vi "DOFreq.vi"(6 "Slot":T1, 8 "error in":errorcluster, 10 "State":string, 11 "CH":string) -> (0 "error out":errorcluster)   [LabVIEW 2013]
uses:
  SystemCode/SysControl/Slot.ctl
  <vilib>/DAQmx/write.llb/DAQmx Write (Digital Bool 1Line 1Point).vi
  SourceCode/GlobalValue.vi
  <vilib>/DAQmx/create/channels.llb/DAQmx Create Channel (DO-Digital Output).vi
  <vilib>/DAQmx/miscellaneous.llb/DAQmx Fill In Error Info.vi
panel:
  out "Line/port":tag="PCI-6229/port0/line0:1"
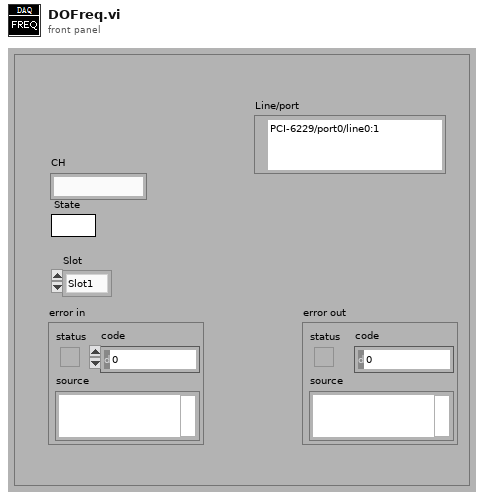
[diagram p1: front panel]
types:
  T1 = typedef "Slot.ctl" = enum16{"Slot1", "Slot2", "Slot3", "Slot4"}
  T2 = typedef "DAQConfig.ctl" = cluster{"DIO":string[][], "AO":string[][], "AI":string[][]}
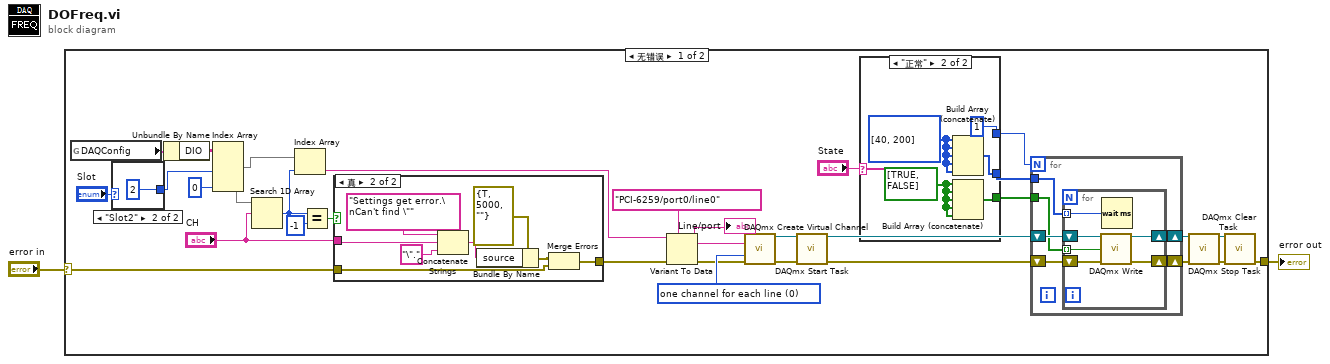
[diagram p0: block diagram]
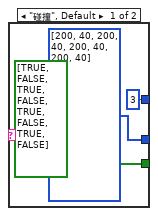
[diagram p2: hidden frame]
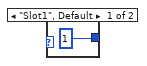
[diagram p3: hidden frame]
diagram:
  n1 = case shown="无错误" "error in" {
    selector: "error in" -> [w22 w65]
    tunnel: [w30 w65] -> w2
    frame No Error {
      w12 = 0 items=["one channel for each line", "one channel for all lines"] ("line grouping")
      n2 = global read "GlobalValue.vi" "DAQConfig"() -> (w19:T2)
      n3 = case shown="\"Slot2\"" "Slot" {
        tunnel: [1 ("索引 (行)") 2 ("索引 (行)")] -> w20
        frame "Slot1", Default {
        }
        frame "Slot2" {
        }
      }
      n4 = Unbundle By Name(w19) -> ("DIO"=w32:string[][])
      n5 = Index Array(array=w32, index (col) #1=w20, index (col) #2=0 ("索引 (列)")) -> (element #1=w24:string[], element #2=w23:string[])  [unwired: 2 in]
      n6 = Search 1D Array(1D array=w23, element="CH") -> (index of element=w29:i32)  [unwired: 1 in]
      n7 = Index Array(array=w24, index=w29) -> (element=w33:string)
      n8 = Equal?(x=w29, y=-1) -> (x = y?=w27:bool)
      n9 = case shown="真" w27 {
        tunnel: "CH" -> [_ w60]
        tunnel: w22 -> [w56 w59]
        tunnel: [w56 w58] -> w26
        frame False {
        }
        frame True {
          n10 = Concatenate Strings("Settings get error.\nCan't find \"" ("message"), w60, "\"." ("string")) -> (w63:string)
          n11 = Bundle By Name(cluster=errorcluster {"status"=TRUE, "code"=5000, "source"=""} ("error in 1 (no error)"), "source"=w63) -> (w62:errorcluster)
          n12 = Merge Errors(w62, w59) -> (w58:errorcluster)
        }
      }
      n13 = Variant To Data(error in=w26, type=tag "PCI-6259/port0/line0" ("lines"), Variant=w33) -> (data=w13:tag, error out=w11:errorcluster)
      "Line/port" <- w13
      n14 = call-poly <vilib>:"DAQmx Create Virtual Channel.vi"("lines"=w13, "line grouping"=w12, "error in"=w11) -> ("task out"=w18:refnum<k21>, "error out"=w17:errorcluster)  [unwired: 11 in]
      n15 = call <vilib>:"DAQmx Start Task.vi"("task/channels in"=w18, "error in"=w17) -> ("task out"=w9:refnum<k21>, "error out"=w10:errorcluster)  [unwired: 12 in]
      n16 = case shown="\"正常\"" "State" {
        tunnel: [u32[] [200, 40, 200, 40, 200, 40, 200, 40] w39] -> w5
        tunnel: [bool[] [TRUE, FALSE, TRUE, FALSE, TRUE, FALSE, TRUE, FALSE] w38] -> w4
        tunnel: [3 1] -> w3
        frame "碰撞", Default {
        }
        frame "正常" {
          w40 = bool[] [TRUE, FALSE]
          w41 = u32[] [40, 200]
          n17 = Build Array (concatenate)(w41, w41, w41, w41, w41) -> (w39:u32[])
          n18 = Build Array (concatenate)(w40, w40, w40, w40, w40) -> (w38:bool[])
        }
      }
      n19 = for {
        N: w3 -> [_]
        shift-right: [w45] -> w8
        shift-left: w10 -> [w47]
        shift-right: [w44] -> w7
        shift-left: w9 -> [w46]
        tunnel: w5 -> [w43]
        tunnel: w4 -> [w42]
        n20 = for {
          tunnel: w42 -> [w51] mode=indexing
          tunnel: w43 -> [w50] mode=indexing
          shift-right: [w49] -> w45
          shift-left: w47 -> [w53]
          shift-right: [w48] -> w44
          shift-left: w46 -> [w52]
          n21 = call-poly <vilib>:"DAQmx Write.vi"("task/channels in"=w52, "data"=w51, "error in"=w53) -> ("task out"=w48:refnum<k21>, "error out"=w49:errorcluster)  [unwired: 10 in, 1 out]
          n22 = Wait (ms)(milliseconds to wait=w50) -> ()  [unwired: 1 out]
        }
      }
      n23 = call <vilib>:"DAQmx Stop Task.vi"("task/channels in"=w7, "error in"=w8) -> ("task out"=w16:refnum<k21>, "error out"=w15:errorcluster)  [unwired: 12 in]
      n24 = call <vilib>:"DAQmx Clear Task.vi"("task in"=w16, "error in"=w15) -> ("error out"=w30:errorcluster)  [unwired: 13 in]
    }
    frame Error {
    }
  }
  "error out" <- w2
